vi "test_ML.vi"() -> ()   [LabVIEW 2020]
uses:
  <vilib>/addons/Machine Learning/Supervised Learning/ml_BP_Terminal Condition.ctl
  <vilib>/addons/Machine Learning/NILabs_MLT.lvlib
panel:
  out "Array":i32[](array[numeric])
  in  "Testing label":i32[](array[numeric])
  in  "Testing data":dbl[][](array[numeric])
  in  "Stopping criteria":T1={"min MSE"=1e-05, "min delta MSE"=1e-08, "min step length"=1e-08, "max iteration"=1000.0}
  in  "Training label":i32[](array[numeric])
  in  "Training data":dbl[][](array[numeric])
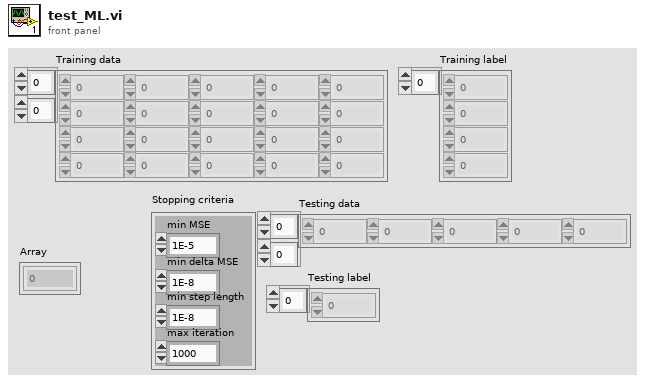
[diagram p1: front panel]
types:
  T1 = typedef "NILabs_MLT.lvlib/ml_BP_Terminal Condition.ctl" = cluster{"min MSE":dbl, "min delta MSE":dbl, "min step length":dbl, "max iteration":dbl}
  T2 = typedef "NILabs_MLT.lvlib/ml_BP_Project.ctl" = cluster{"Training Data":T3, "Normalize Info":T4, "3-layer NN":T5, "Ternimal Condition":T1}
  T3 = typedef "NILabs_MLT.lvlib/ml_BP_Data.ctl" = cluster{"dim in":i32, "dim out":i32, "# samples":i32, "Input":dbl[][], "Output":dbl[][]}
  T4 = typedef "NILabs_MLT.lvlib/ml_BP_Normalize Data.ctl" = cluster{"input min":dbl[], "input max":dbl[], "output min":dbl[], "output max":dbl[]}
  T5 = typedef "NILabs_MLT.lvlib/ml_BP_3layer Feedforward.ctl" = cluster{"# input neuron ":i32, "# hidden neuron":i32, "# output neuron":i32, "Weight (I->H)":dbl[][], "Weight (H->O)":dbl[][], "Output":dbl[][], "Hidden Out":dbl[][], "Derivation Output":dbl[][], "Derivation Hidden":dbl[][], "dw (I->H)":dbl[][], "dw (H->O)":dbl[][]}
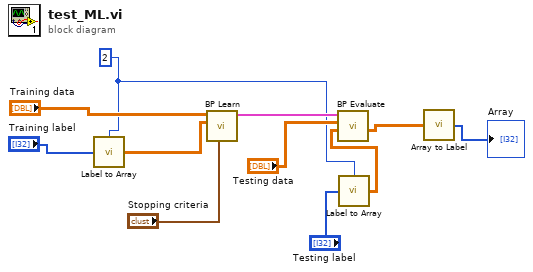
[diagram p0: block diagram]
diagram:
  w2 = 2
  n1 = call <vilib>:"Label to Array.vi"("Classes"="Training label", "# of classes"=w2) -> ("Array"=w7:dbl[][])
  n2 = call <vilib>:"BP Learn.vi"("Stopping Criteria"="Stopping criteria", "Training outputs"=w7, "Training data samples"="Training data") -> ("BP Project"=w11:T2)  [unwired: 5 in, 3 out]
  n3 = call <vilib>:"Label to Array.vi"("Classes"="Testing label", "# of classes"=w2) -> ("Array"=w3:dbl[][])
  n4 = call <vilib>:"BP Evaluate.vi"("Test outputs"=w3, "Test data samples"="Testing data", "BP Project"=w11) -> ("NN outputs"=w10:dbl[][])  [unwired: 4 in, 4 out]
  n5 = call <vilib>:"Array to Label.vi"("Array"=w10) -> ("Classes"=→"Array":i32[])
